vi "CCE MGLD PMJD PF SubVI07.vi"(3 "B":u8, 4 "G":u8, 5 "R":u8) -> (2 "RGB2GRAY":u8)   [LabVIEW 2020]
doc: "Ceballos Conde Emanuel Meneses Gutiérrez Luis David Pineda Méndez Job Daniel 4MV6 Sistemas de visión artificial 2022/1 \nEste VI realizar la escala de grises a partir de los valores de la funcion de MATLAB rgbtogray"
panel:
  out "Color 2":u32(colorbox)
  out "Color":u32(colorbox)
  # "Ceballos Conde Emanuel   -  Meneses Gutiérrez Luis David   -  Pineda Méndez Job Daniel 4MV6 Sistemas de visión artificial  2022/1             SubVI07"
  # "RGB2GRAY"
  # "RGB"
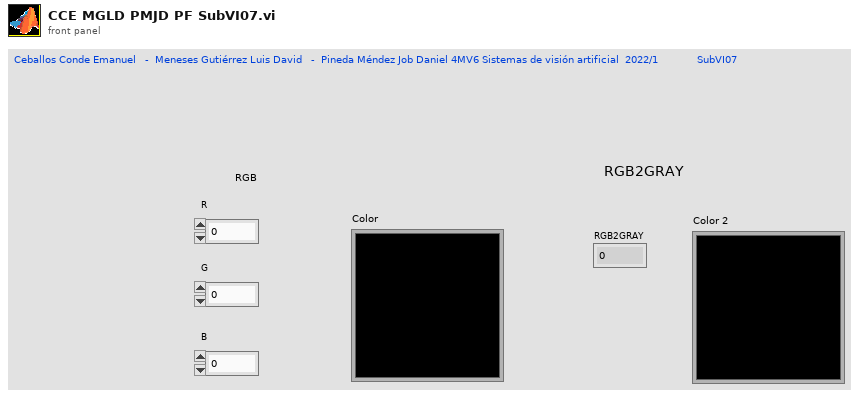
[diagram p1: front panel]
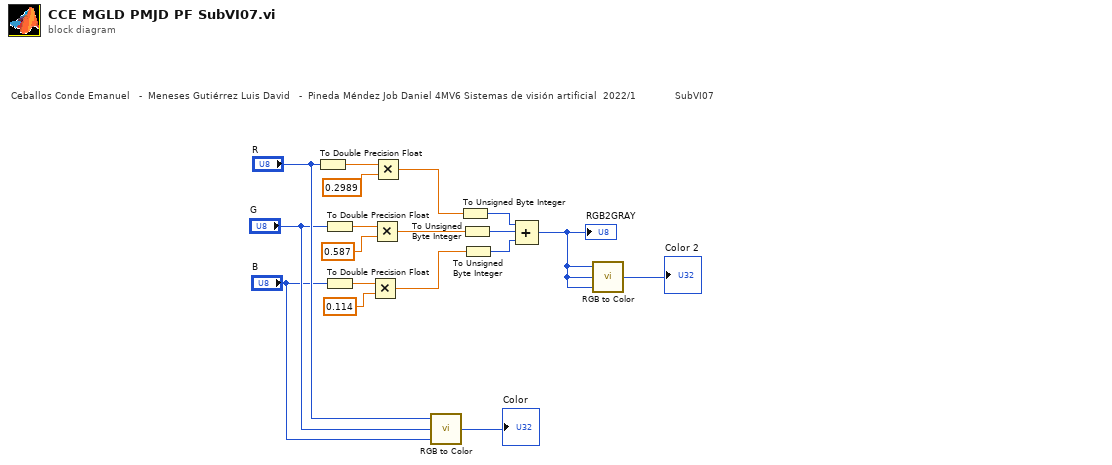
[diagram p0: block diagram]
diagram:
  # "Ceballos Conde Emanuel   -  Meneses Gutiérrez Luis David   -  Pineda Méndez Job Daniel 4MV6 Sistemas de visión artificial  2022/1             SubVI07"
  n1 = To Double Precision Float(number="R") -> (double precision float=w11:dbl)
  n2 = To Double Precision Float(number="G") -> (double precision float=w10:dbl)
  n3 = To Double Precision Float(number="B") -> (double precision float=w9:dbl)
  n4 = Multiply(x=w9, y=0.114) -> (x*y=w3:dbl)
  n5 = Multiply(x=w10, y=0.587) -> (x*y=w4:dbl)
  n6 = Multiply(x=w11, y=0.2989) -> (x*y=w5:dbl)
  n7 = call <vilib>:"RGB to Color.vi"("B"="B", "G"="G", "R"="R") -> ("Color"=→"Color":u32)
  n8 = To Unsigned Byte Integer(number=w5) -> (unsigned 8bit integer=w14:u8)
  n9 = To Unsigned Byte Integer(number=w4) -> (unsigned 8bit integer=w13:u8)
  n10 = To Unsigned Byte Integer(number=w3) -> (unsigned 8bit integer=w12:u8)
  n11 = Compound Arithmetic op=ADD(w14, w13, w12) -> (w1:u8)
  "RGB2GRAY" <- w1
  n12 = call <vilib>:"RGB to Color.vi"("B"=w1, "G"=w1, "R"=w1) -> ("Color"=→"Color 2":u32)
